vi "Heat1D_Iteration Solve.vi"(0 "U(n)":dbl[](array[numeric]), 1 "Coeff Array":dbl[](array[numeric]), 2 "F(x,t)":dbl[][](array[numeric]), 3 "step":i32, 5 "L":dbl[](array[numeric]), 7 "U":T1, 9 "Pivot":i32[](array[numeric]), 11 "BC Type":i32, 12 "Left BC":dbl, 13 "Right BC":dbl) -> (4 "U(n+1)":dbl[](array[numeric]))   [LabVIEW 2017, in "NI_PDE.lvlib"]
uses:
  <vilib>/gmath/NI_PDE.lvlib
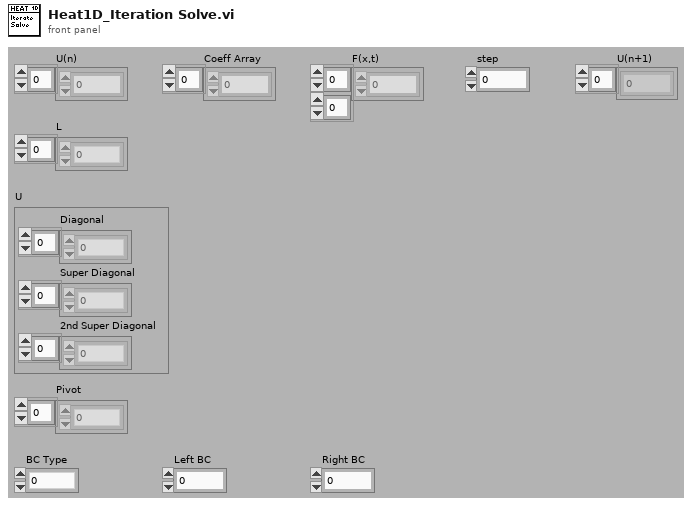
[diagram p1: front panel]
types:
  T1 = cluster{"Diagonal":dbl[], "Super Diagonal":dbl[], "2nd Super Diagonal":dbl[]}
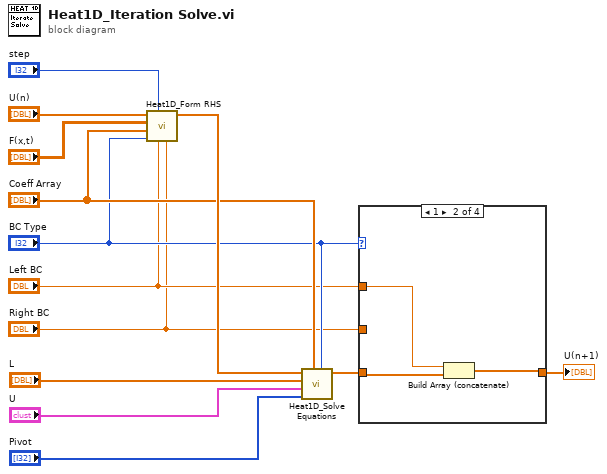
[diagram p0: block diagram]
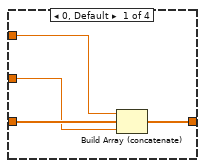
[diagram p2: hidden frame]
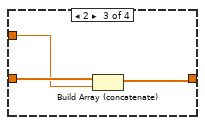
[diagram p3: hidden frame]
diagram:
  n1 = call <vilib>:"Heat1D_Form RHS.vi"("Right BC"="Right BC", "Left BC"="Left BC", "step"="step", "BC Type"="BC Type", "Coeff Array"="Coeff Array", "F(x,t)"="F(x,t)", "U(n)"="U(n)") -> ("RHS"=w12:dbl[])  [unwired: 4 in]
  n2 = call <vilib>:"Heat1D_Solve Equations.vi"("BC Type"="BC Type", "Coeff Array"="Coeff Array", "Pivot"="Pivot", "U"="U", "L"="L", "RHS"=w12) -> ("Solution Vector"=w3:dbl[])  [unwired: 5 out]
  n3 = case shown="1" "BC Type" {
    tunnel: w3 -> [w17 w19 w23 w24]
    tunnel: "Left BC" -> [w16 w20 _ _]
    tunnel: "Right BC" -> [w15 _ w22 _]
    tunnel: [w14 w18 w21 w24] -> w2
    frame 0, Default {
      n4 = Build Array (concatenate)(w16, w17, w15) -> (w14:dbl[])
    }
    frame 1 {
      n5 = Build Array (concatenate)(w20, w19) -> (w18:dbl[])
    }
    frame 2 {
      n6 = Build Array (concatenate)(w23, w22) -> (w21:dbl[])
    }
    frame 3 {
    }
  }
  "U(n+1)" <- w2
